vi "test_imaqdx_basic.vi"() -> ()   [LabVIEW 2019]
uses:
  <vilib>/vision/driver/IMAQdx.llb/IMAQdx Buffer Number Mode.ctl
  <vilib>/vision/driver/NI_Vision_Acquisition_Software.lvlib
  <vilib>/vision/NI_Vision_Development_Module.lvlib
panel:
  out "error out 2":errorcluster
  out "error out":errorcluster
  out "Image Pixels (U8) 2":u8[][](array[numeric])
  in  "Color Plane":i32(ring)=1 items=["Red", "Green", "Blue", "Hue", "Saturation", "Luminance", "Value", "Intensity"]
  out "Image Pixels (U8)":u8[][](array[numeric])
  in  "Color Mode":u16(ring) items=["RGB", "HSL", "HSV", "HSI"]
  in  "Camera Name":refnum<k21>="cam0" caption="IMAQdx Session"
  in  "Stop":bool
  out "Image":T1(plugin-control)
  out "Buffer Number":u32=195
  out "Acquisition Frame Rate":dbl=33.36604514229637 format="%.1f"
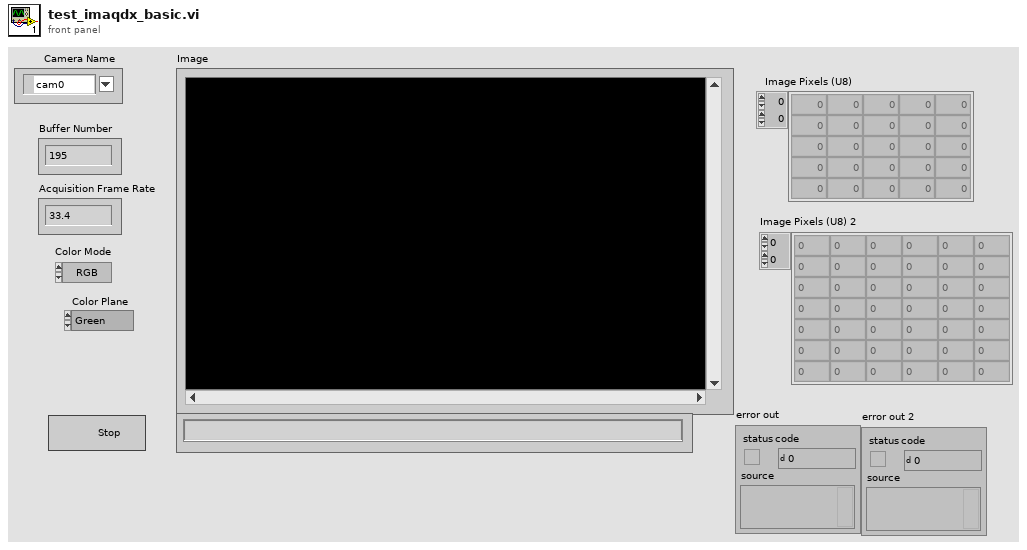
[diagram p1: front panel]
types:
  T1 = typedef "IMAQ Image.ctl" = refnum<image>
  T2 = typedef "Image Type" = u32
  T3 = typedef "IMAQdx.ctl" = refnum<k21>
  T4 = typedef "NI_Vision_Acquisition_Software.lvlib/IMAQdx Buffer Number Mode.ctl" = enum32{"Next", "Last", "Buffer Number", "Every", "Last New"}
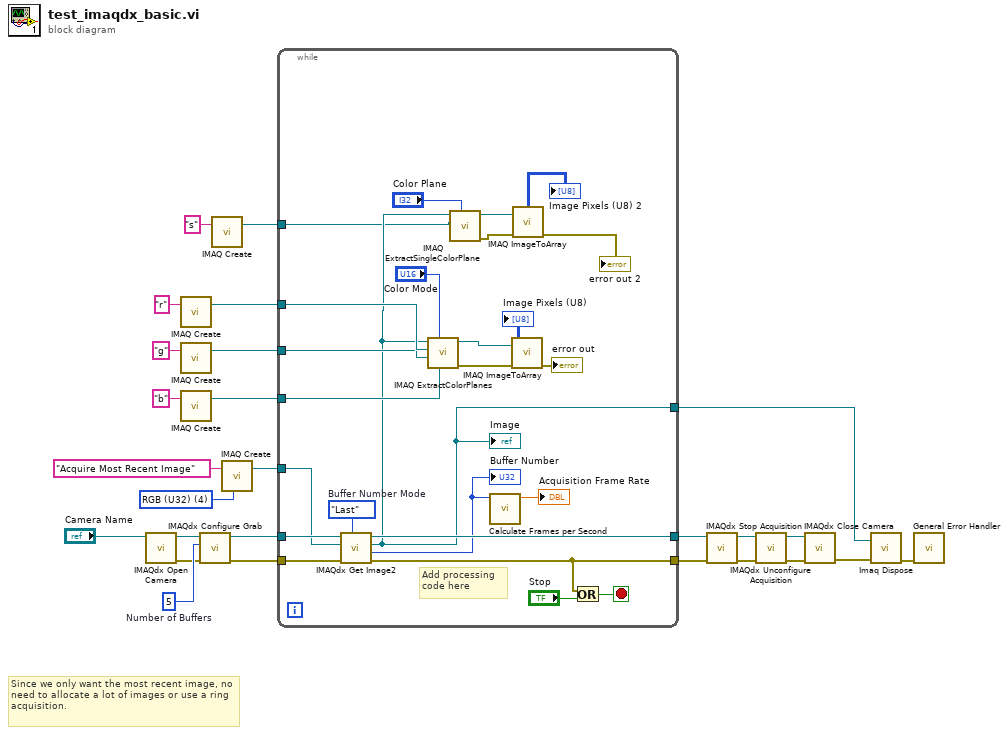
[diagram p0: block diagram]
diagram:
  w3 = T2 4 items=["Grayscale (U8)", "Grayscale (I16)", "Grayscale (SGL)", "Complex (CSG)", "RGB (U32)", "HSL (U32)", "RGB (U64)", "Grayscale (U16)"] ("Image Type")
  w13 = u32 5  # Number of Buffers
  # "Since we only want the most recent image, no need to allocate a lot of images or use a ring acquisition."
  n1 = call <vilib>:"IMAQdx Open Camera.vi"("Session In"="Camera Name") -> ("error out"=w12:errorcluster, "Session Out"=w14:T3)  [unwired: 2 in, 7 out]
  n2 = call "IMAQ Create"("Image Name"="r") -> ("New Image"=w6:T1)  [unwired: 3 in, 2 out]
  n3 = call "IMAQ Create"("Image Name"="g") -> ("New Image"=w5:T1)  [unwired: 3 in, 2 out]
  n4 = call "IMAQ Create"("Image Name"="b") -> ("New Image"=w4:T1)  [unwired: 3 in, 2 out]
  n5 = call <vilib>:"IMAQdx Configure Grab.vi"("error in"=w12, "Number of Buffers"=w13, "Session In"=w14) -> ("error out"=w10:errorcluster, "Session Out"=w11:T3)  [unwired: 7 in]
  n6 = call "IMAQ Create"("Image Name"="s") -> ("New Image"=w1:T1)  [unwired: 3 in, 2 out]
  n7 = call "IMAQ Create"("Image Name"="Acquire Most Recent Image", "Image Type"=w3) -> ("New Image"=w26:T1)  [unwired: 2 in, 2 out]
  n8 = while {
    tunnel: [w45] -> w23
    tunnel: w10 -> [w49]
    tunnel: w11 -> [w50]
    tunnel: [w42] -> w24
    tunnel: w26 -> [w48]
    tunnel: [w28] -> w15
    tunnel: w6 -> [w41]
    tunnel: w5 -> [w40]
    tunnel: w4 -> [w39]
    tunnel: w1 -> [w27]
    stop <- w51 stop-if-true
    w47 = IMAQdx_Buffer_Number_Mode."Last"  # Buffer Number Mode
    # "Add processing code here"
    n9 = call <vilib>:"IMAQdx Get Image2.vi"("Buffer Number Mode (Next)"=w47, "error in"=w49, "Image In"=w48, "Session In"=w50) -> ("error out"=w42:errorcluster, "Buffer Number Out"=w44:u32, "Image Out"=w28:T1, "Session Out"=w45:T3)  [unwired: 4 in]
    "Image" <- w28
    "Buffer Number" <- w44
    n10 = call "IMAQ ExtractColorPlanes"("Blue or Luma or Val or Inten Plane"=w39, "Color Mode"="Color Mode", "Green or Sat Plane"=w40, "Red or Hue Plane"=w41, "Image Src"=w28) -> ("error out"=w32:errorcluster, "Red or Hue Plane out"=w37:T1)  [unwired: 3 in, 2 out]
    n11 = call "IMAQ ExtractSingleColorPlane"("Color Plane"="Color Plane", "Image Dst"=w27, "Image Src"=w28) -> ("error out"=w30:errorcluster, "Image Dst Out"=w34:T1)  [unwired: 7 in]
    n12 = call <vilib>:"Calculate Frames per Second.vi"("Buffer Number"=w44) -> ("Acquired Frames/s"=→"Acquisition Frame Rate":dbl)  [unwired: 8 in, 2 out]
    n13 = call "IMAQ ImageToArray"("error in (no error)"=w32, "Image"=w37) -> ("error out"=→"error out":errorcluster, "Image Pixels (U8)"=→"Image Pixels (U8)":u8[][])  [unwired: 2 in, 3 out]
    n14 = call "IMAQ ImageToArray"("error in (no error)"=w30, "Image"=w34) -> ("error out"=→"error out 2":errorcluster, "Image Pixels (U8)"=→"Image Pixels (U8) 2":u8[][])  [unwired: 2 in, 3 out]
    n15 = Or(x=w42, y="Stop") -> (x .or. y?=w51:bool)
  }
  n16 = call <vilib>:"IMAQdx Stop Acquisition.vi"("error in"=w24, "Session In"=w23) -> ("error out"=w19:errorcluster, "Session Out"=w20:T3)  [unwired: 8 out]
  n17 = call <vilib>:"IMAQdx Unconfigure Acquisition.vi"("error in"=w19, "Session In"=w20) -> ("error out"=w22:errorcluster, "Session Out"=w21:T3)  [unwired: 8 out]
  n18 = call <vilib>:"IMAQdx Close Camera.vi"("error in"=w22, "Session In"=w21) -> ("error out"=w18:errorcluster)  [unwired: 9 out]
  n19 = call "Imaq Dispose"("Image"=w15, "error in (no error)"=w18) -> ("error out"=w17:errorcluster)  [unwired: 4 in]
  n20 = call <vilib>:"General Error Handler.vi"("error in (no error)"=w17) -> ()  [unwired: 2 in, 13 out]
